vi "test_memory_leak.vi"() -> ()   [LabVIEW 2015]
panel:
  out "Numeric":i32
  in  "Clean":bool
  in  "Add":bool
  in  "stop":bool
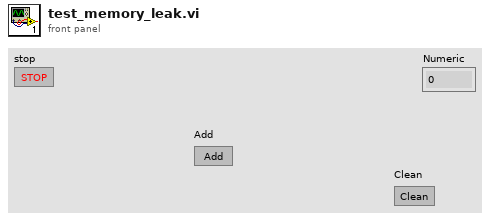
[diagram p1: front panel]
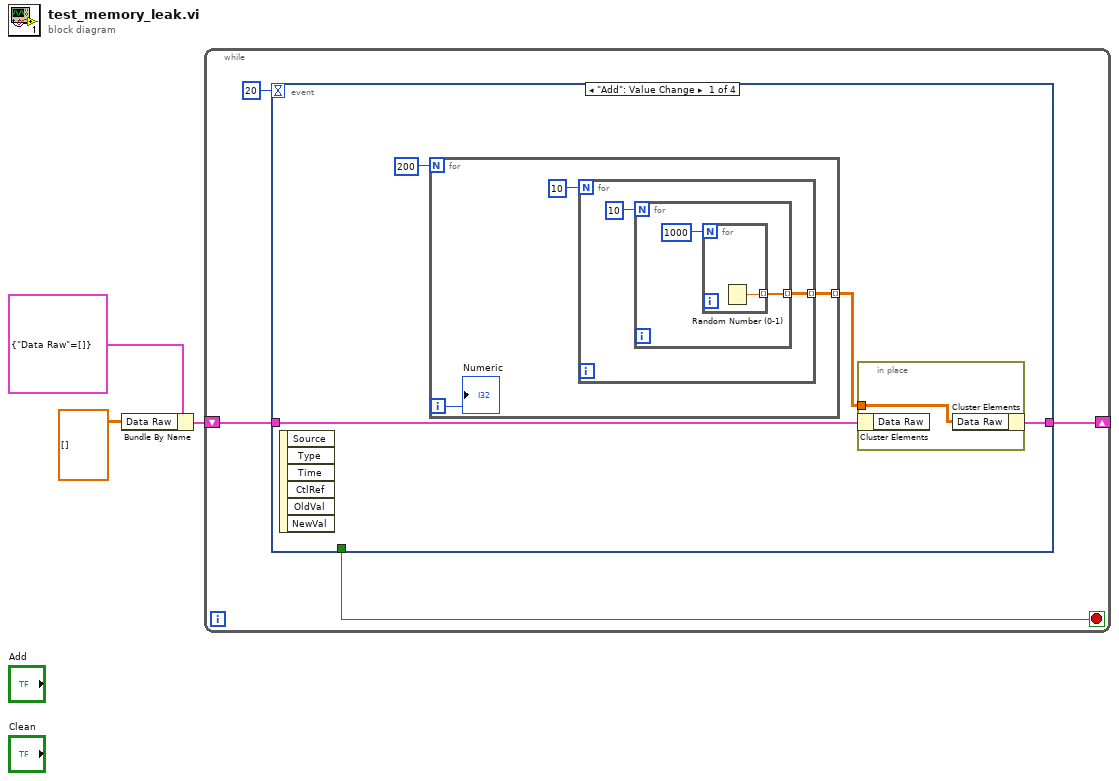
[diagram p0: block diagram]
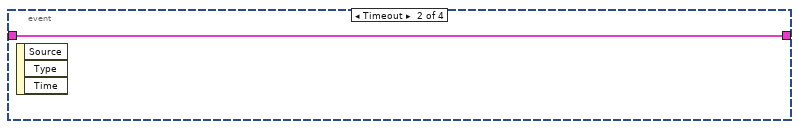
[diagram p2: hidden frame]
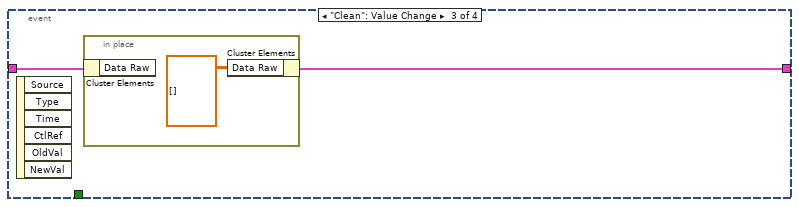
[diagram p3: hidden frame]
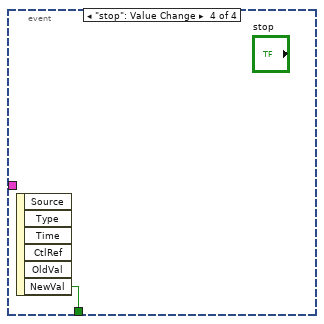
[diagram p4: hidden frame]
diagram:
  n1 = Bundle By Name(cluster=cluster{"Data Raw":dbl[][][][]} {"Data Raw"=[]}, "Data Raw"=dbl[][][][] []) -> (w1:cluster{"Data Raw":dbl[][][][]})
  n2 = while {
    shift-right: [w6] -> _
    shift-left: w1 -> [w5]
    stop <- w4 stop-if-true
    n3 = event shown="[0] \"Add\": Value Change" {
      selector: _ -> [_ _ _ _]
      dyn-events: _ -> [_ _ _ _]
      timeout: 20 -> [_ _ _ _]
      tunnel: [w10 w21 w22 _] -> w6
      tunnel: w5 -> [w11 w21 w23 _]
      tunnel: [_ _ _ w25] -> w4
      event "Add": Value Change {
        n4 = event-data() -> ()  [unwired: 1 in, 6 out]
        n5 = for {
          N: 200 -> [_]
          tunnel: [w14] -> w8 mode=indexing
          i -> [w12]
          n6 = for {
            N: 10 -> [_]
            tunnel: [w16] -> w14 mode=indexing
            n7 = for {
              N: 10 -> [_]
              tunnel: [w18] -> w16 mode=indexing
              n8 = for {
                N: 1000 -> [_]
                tunnel: [w19] -> w18 mode=indexing
                n9 = Random Number (0-1)() -> (number: 0 to 1=w19:dbl)
              }
            }
          }
          "Numeric" <- w12
        }
        n10 = in-place {
          in-place-border: w8 -> [w20]
          n11 = in-place-cluster #1(w11) -> ()  [unwired: 1 out]
          n12 = in-place-cluster #1("Data Raw"=w20) -> (w10:cluster{"Data Raw":dbl[][][][]})
        }
      }
      event Timeout {
        n13 = event-data() -> ()  [unwired: 1 in, 3 out]
      }
      event "Clean": Value Change {
        n14 = event-data() -> ()  [unwired: 1 in, 6 out]
        n15 = in-place {
          n16 = in-place-cluster #2(w23) -> ()  [unwired: 1 out]
          n17 = in-place-cluster #2("Data Raw"=dbl[][][][] []) -> (w22:cluster{"Data Raw":dbl[][][][]})
        }
      }
      event "stop": Value Change {
        n18 = event-data() -> ("NewVal"=w25:bool)  [unwired: 1 in, 5 out]
      }
    }
  }
